vi "Read Serial Data.vi"(8 "error in (no error)":errorcluster, 10 "Maximum Characters (32)":i32=32, 11 "VISA resource name":refnum<visa-resource-name>) -> (0 "error out":errorcluster, 2 "Serial Data":string, 3 "VISA resource name out":refnum<visa-resource-name>)   [LabVIEW 2019, in "Keithley 2600 Series.lvlib"]
doc: "Returns data from the serial port. \n\n<b>Note:</b>\nThis VI is not available on the model 2606B."
uses:
  Keithley 2600 Series.lvlib
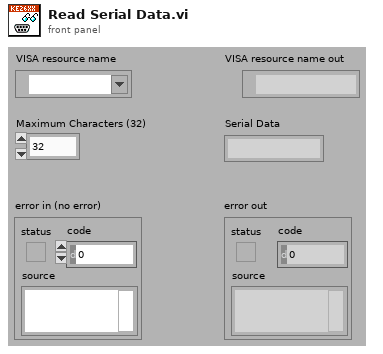
[diagram p1: front panel]
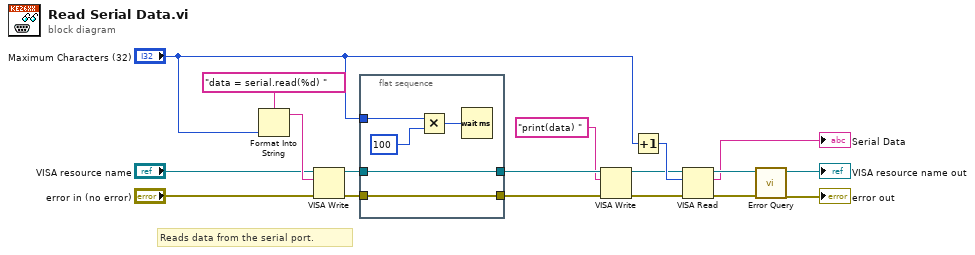
[diagram p0: block diagram]
diagram:
  # "Reads data from the serial port."
  n1 = Format Into String(format string="data = serial.read(%d) ", "Maximum Characters (32)") -> (resulting string=w17:string)  [unwired: 2 in, 1 out]
  n2 = VISA Write(VISA resource name="VISA resource name", write buffer=w17, error in (no error)="error in (no error)") -> (VISA resource name out=w8:refnum<visa-resource-name>, error out=w7:errorcluster)  [unwired: 1 out]
  n3 = flat-sequence {
    tunnel: w8 -> [w23]
    tunnel: [w23] -> w6
    tunnel: w7 -> [w22]
    tunnel: [w22] -> w4
    tunnel: "Maximum Characters (32)" -> [w19]
    frame #0 {
      n4 = Multiply(x=w19, y=100) -> (x*y=w20:i32)
      n5 = Wait (ms)(milliseconds to wait=w20) -> ()  [unwired: 1 out]
    }
  }
  n6 = VISA Write(VISA resource name=w6, write buffer="print(data) ", error in (no error)=w4) -> (VISA resource name out=w5:refnum<visa-resource-name>, error out=w3:errorcluster)  [unwired: 1 out]
  n7 = Increment(x="Maximum Characters (32)") -> (x+1=w9:i32)
  n8 = VISA Read(VISA resource name=w5, byte count=w9, error in (no error)=w3) -> (VISA resource name out=w12:refnum<visa-resource-name>, read buffer=→"Serial Data":string, error out=w11:errorcluster)  [unwired: 1 out]
  n9 = call "Error Query.vi"("error in (no error)"=w11, "VISA resource name"=w12) -> ("error out"=→"error out":errorcluster, "VISA resource name out"=→"VISA resource name out":refnum<visa-resource-name>)  [unwired: 6 in, 2 out]
